vi "Initialise Checkerboard Floor.vi"(8 "error in (no error)":errorcluster, 10 "Number Of Squares Per Side":i32=8, 11 "Resource Directory":path) -> (0 "error out":errorcluster, 3 "Checkerboard Floor":T1[](array[typedef]) {"Triangles"."Vertex 3"."UV"."v" min=0 max=1 step=0.1; "Triangles"."Vertex 3"."UV"."u" min=0 max=1 step=0.1; "Triangles"."Vertex 2"."UV"."v" min=0 max=1 step=0.1; "Triangles"."Vertex 2"."UV"."u" min=0 max=1 step=0.1; "Triangles"."Vertex 1"."UV"."v" min=0 max=1 step=0.1; "Triangles"."Vertex 1"."UV"."u" min=0 max=1 step=0.1})   [LabVIEW 2020, in "Application.lvlib" / "Scene.lvclass"]
uses:
  Scene.lvclass
  Scene.lvclass/Scene.ctl
  FPGA/Libraries/3D/3D (FPGA).lvlib
  FPGA/Libraries/3D/Vector 3D.ctl
  FPGA/Libraries/3D/Transform.ctl
  FPGA/Libraries/3D/Object.ctl
  FPGA/Libraries/Raster/UV.ctl
  FPGA/Libraries/Raster/Raster (FPGA).lvlib
  FPGA/Libraries/3D/Vertex.ctl
  FPGA/Libraries/3D/Triangle.ctl
  FPGA/Libraries/Raster/Rectangle Dimensions.ctl
  FPGA/Libraries/Raster/Texture.ctl
  FPGA/Libraries/3D/Material.ctl
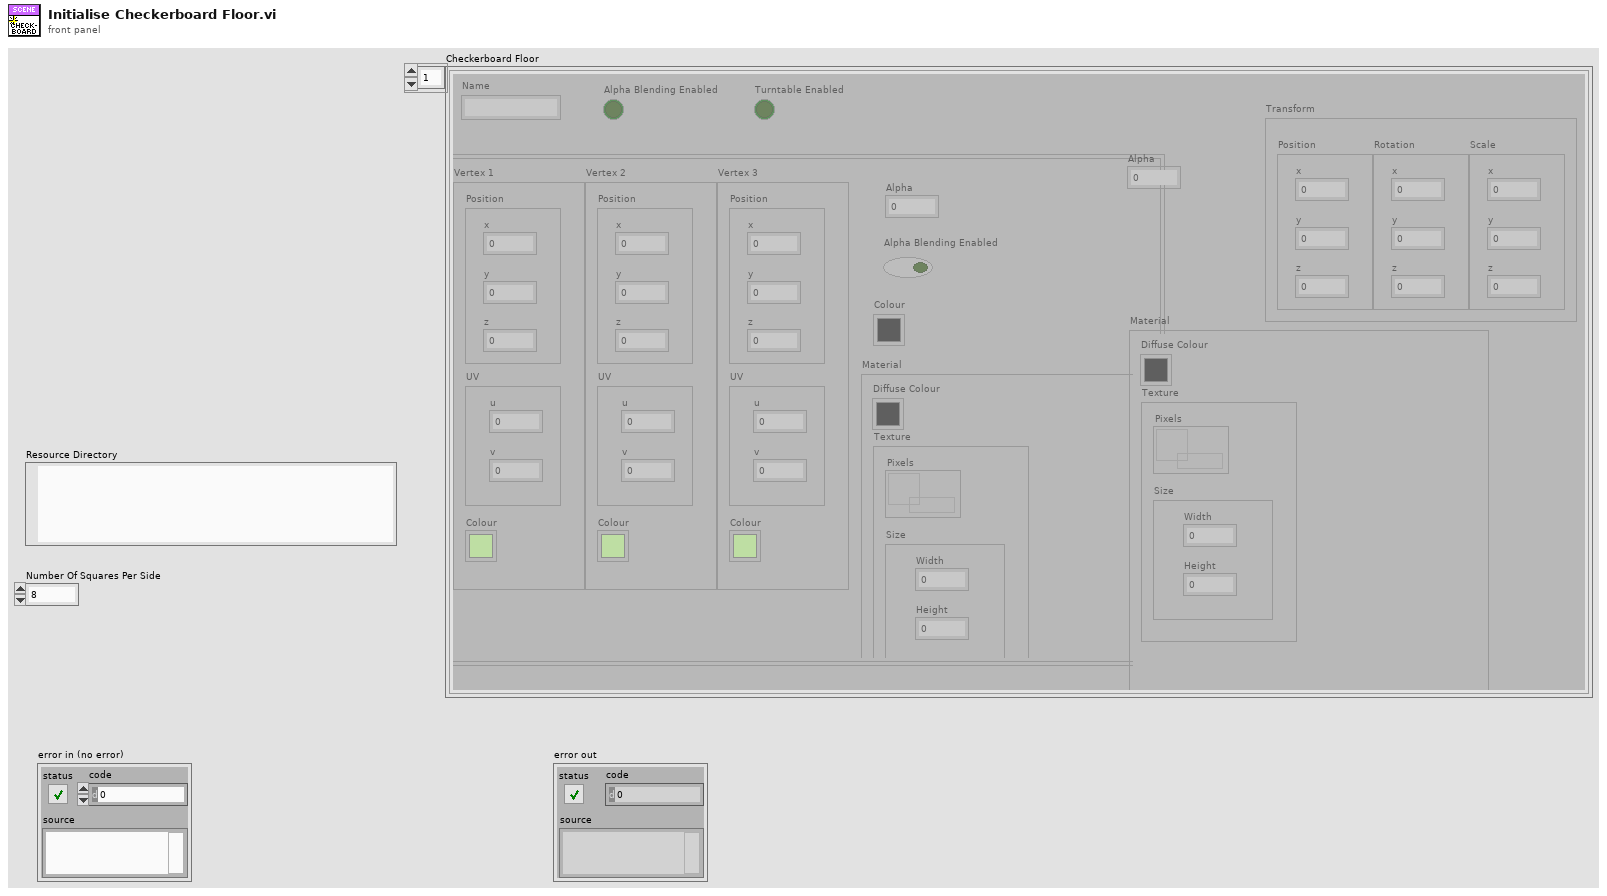
[diagram p1: front panel]
types:
  T1 = typedef "3D (FPGA).lvlib/Object.ctl" = cluster{"Triangles":T2[], "Transform":T9, "Name":string, "Alpha Blending Enabled":bool, "Alpha":dbl, "Turntable Enabled":bool, "Material":T6}
  T2 = typedef "3D (FPGA).lvlib/Triangle.ctl" = cluster{"Vertex 1":T3, "Vertex 2":T3, "Vertex 3":T3, "Alpha":dbl, "Alpha Blending Enabled":bool, "Colour":u32, "Material":T6}
  T3 = typedef "3D (FPGA).lvlib/Vertex.ctl" = cluster{"Position":T4, "UV":T5, "Colour":u32}
  T4 = typedef "3D (FPGA).lvlib/Vector 3D.ctl" = cluster{"x":sgl, "y":sgl, "z":sgl}
  T5 = typedef "Raster (FPGA).lvlib/UV.ctl" = cluster{"u":sgl, "v":sgl}
  T6 = typedef "3D (FPGA).lvlib/Material.ctl" = cluster{"Diffuse Colour":u32, "Texture":T7}
  T7 = typedef "Raster (FPGA).lvlib/Texture.ctl" = cluster{"Pixels":refnum<data-value>, "Size":T8}
  T8 = typedef "Raster (FPGA).lvlib/Rectangle Dimensions.ctl" = cluster{"Width":u32, "Height":u32}
  T9 = typedef "3D (FPGA).lvlib/Transform.ctl" = cluster{"Position":T4, "Rotation":T4, "Scale":T4}
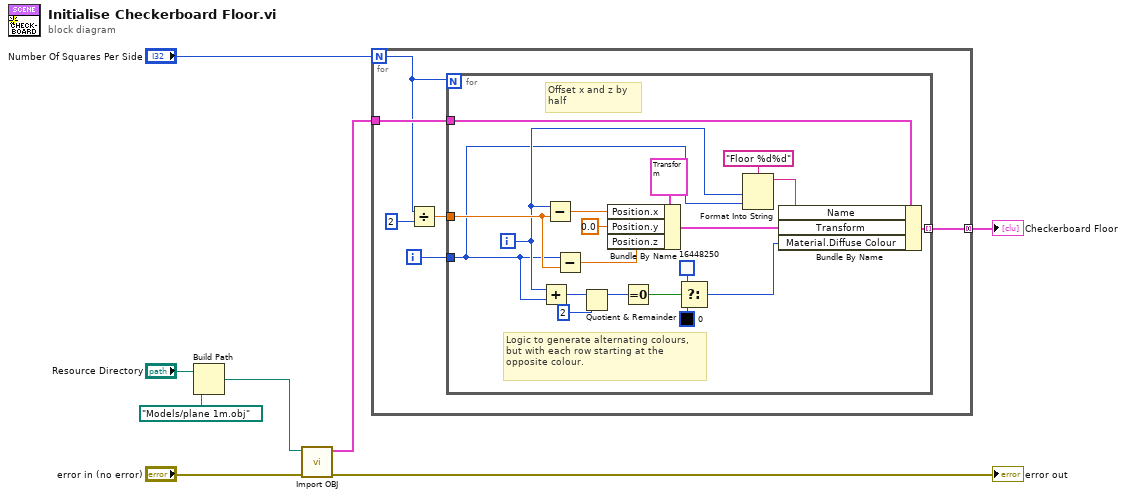
[diagram p0: block diagram]
diagram:
  n1 = Build Path(base path="Resource Directory", name or relative path=path "Models/plane 1m.obj") -> (appended path=w1:path)
  n2 = call "Import OBJ.vi"("error in (no error)"="error in (no error)", "Object"=w1) -> ("error out"=→"error out":errorcluster, "Object"=w6:T1)  [unwired: 8 in]
  n3 = for {
    N: "Number Of Squares Per Side" -> [w11]
    tunnel: w6 -> [w14]
    tunnel: [w13] -> w5 mode=concatenating
    i -> [w12]
    n4 = Divide(x=w11, y=2) -> (x/y=w9:dbl)
    n5 = for {
      N: w11 -> [_]
      tunnel: w14 -> [w30]
      tunnel: [w29] -> w13 mode=indexing
      tunnel: w12 -> [w16]
      tunnel: w9 -> [w20]
      i -> [w17]
      # "Logic to generate alternating colours, but with each row starting at the opposite colour."
      # "Offset x and z by half"
      n6 = Add(x=w17, y=w16) -> (x+y=w26:i32)
      n7 = Subtract(x=w17, y=w20) -> (x-y=w22:dbl)
      n8 = Subtract(x=w16, y=w20) -> (x-y=w21:dbl)
      n9 = Quotient & Remainder(x=w26, y=2) -> (x-y*floor(x/y)=w24:i32)  [unwired: 1 out]
      n10 = Bundle By Name(cluster=T9 {"Position"={"x"=2.0, "y"=1.0, "z"=-5.0}, "Rotation"={"x"=0.0, "y"=0.0, "z"=0.0}, "Scale"={"x"=0.0, "y"=0.0, "z"=0.0}} ("Transform"), "Position.x"=w22, "Position.y"=sgl 0.0, "Position.z"=w21) -> (w32:T9)
      n11 = Equal To 0?(x=w24) -> (x = 0?=w23:bool)
      n12 = Select(t=u32 16448250 ("Diffuse Colour"), s=w23, f=u32 0 ("Diffuse Colour")) -> (s? t:f=w15:u32)
      n13 = Format Into String(format string="Floor %d%d" ("Name"), w17, w16) -> (resulting string=w18:string)  [unwired: 2 in, 1 out]
      n14 = Bundle By Name(cluster=w30, "Name"=w18, "Transform"=w32, "Material.Diffuse Colour"=w15) -> (w29:T1)
    }
  }
  "Checkerboard Floor" <- w5
